vi "Startup.vi"(5 "DAQ":refnum<class "DAQ.lvclass">, 6 "DataQueues":refnum<class "DataQueues.lvclass">, 7 "Application":refnum<class "Application.lvclass">, 8 "error in (no error)":errorcluster, 9 "Config":refnum<class "Config.lvclass">=refnum, 10 "Sequencer":refnum<class "Sequencer.lvclass">=refnum, 11 "LogEngine":refnum<class "LogEngine.lvclass">) -> (0 "error out":errorcluster, 3 "LogEngine.lvclass":refnum<class "LogEngine.lvclass">)   [LabVIEW 2022 SP3, in "LogEngine.lvclass"]
doc: "Developed by Kevin Thompson\nkevin@thompsonengineering.net\n\nCopyright 2018-2020\nThompson Engineering, LLC"
uses:
  LogEngine.lvclass
  LogEngine.lvclass/LogEngine.ctl
  Data Types/TD Logger State Data--cluster.ctl
  Data Types/TD Logger State--enum.ctl
  Support/DataQueues/DataQueues.lvclass
  DAQ/DAQ.lvclass
  Data Types/Dependency--cluster.ctl
  Config/Config.lvclass
  Application/Application.lvclass
  Sequencer/Sequencer.lvclass
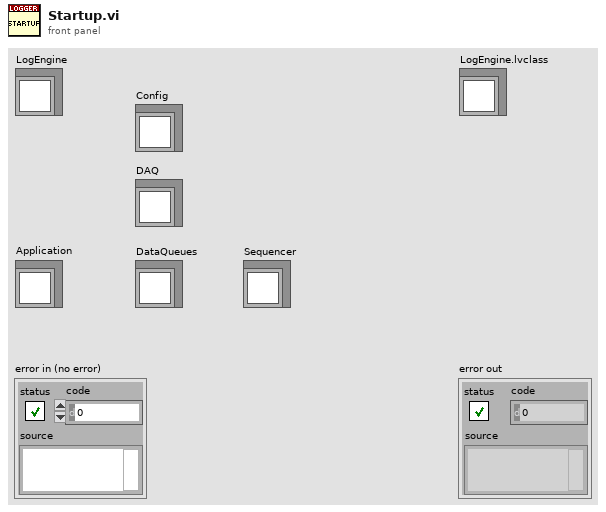
[diagram p1: front panel]
types:
  T1 = typedef "LogEngine.lvclass/Dependency--cluster.ctl" = cluster{"DataQueues":refnum<class "DataQueues.lvclass">, "DAQ":refnum<class "DAQ.lvclass">}
  T2 = typedef "LogEngine.lvclass/TD Logger State Data--cluster.ctl" = cluster{"Logger State":T3, "TDMS Logging State":T3, "LogFile path":path, "TDMS File path":path, "vData":variant}
  T3 = typedef "LogEngine.lvclass/TD Logger State--enum.ctl" = enum16{"Unknown", "Logging", "NotLogging", "Error"}
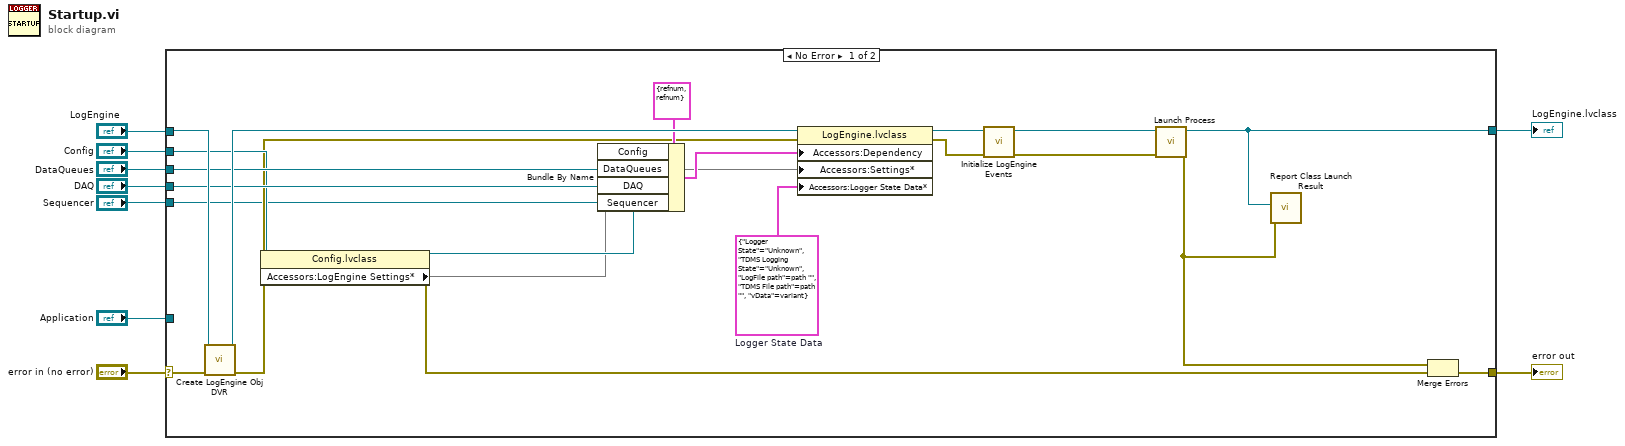
[diagram p0: block diagram]
diagram:
  n1 = case shown="No Error" "error in (no error)" {
    selector: "error in (no error)" -> [w28 w32]
    tunnel: [w30 w32] -> w8
    tunnel: [w12 w31] -> w6
    tunnel: "LogEngine" -> [w27 w31]
    tunnel: "Application" -> [_ _]
    tunnel: "DataQueues" -> [w20 _]
    tunnel: "DAQ" -> [w19 _]
    tunnel: "Config" -> [w17 _]
    tunnel: "Sequencer" -> [w10 _]
    frame No Error {
      w22 = T2 {"Logger State"=enum."Unknown", "TDMS Logging State"=enum."Unknown", "LogFile path"=path "", "TDMS File path"=path "", "vData"=variant}  # Logger State Data
      n2 = call "Create LogEngine Obj DVR.vi"("error in (no error)"=w28, "LogEngine.lvclass"=w27) -> ("error out"=w14:errorcluster, "LogEngine.lvclass"=w26:refnum<class "LogEngine.lvclass">)  [unwired: 8 in]
      n3 = property class="Config.lvclass"(reference=w17, error in=w14) -> (reference out=w16:refnum<class "Config.lvclass">, error out=w13:errorcluster, "Accessors:LogEngine Settings*"=w15)
      n4 = Bundle By Name(cluster=T1 {"DataQueues"=refnum, "DAQ"=refnum} ("Dependency"), "Config"=w16, "DataQueues"=w20, "DAQ"=w19, "Sequencer"=w10) -> (w18:T1)
      n5 = property class="LogEngine.lvclass"(reference=w26, error in=w14, "Accessors:Dependency"=w18, "Accessors:Settings*"=w15, "Accessors:Logger State Data*"=w22) -> (reference out=w25:refnum<class "LogEngine.lvclass">, error out=w29:errorcluster)
      n6 = call "Initialize LogEngine Events.vi"("error in (no error)"=w29, "LogEngine.lvclass"=w25) -> ("error out"=w23:errorcluster, "LogEngine.lvclass"=w24:refnum<class "LogEngine.lvclass">)  [unwired: 8 in]
      n7 = call "Launch Process.vi"("error in (no error)"=w23, "LogEngine.lvclass"=w24) -> ("error out"=w11:errorcluster, "LogEngine.lvclass"=w12:refnum<class "LogEngine.lvclass">)  [unwired: 8 in]
      n8 = call "Report Class Launch Result.vi"("Object"=w12, "error in (no error)"=w11) -> ()  [unwired: 8 in, 1 out]
      n9 = Merge Errors(w11, w13) -> (w30:errorcluster)
    }
    frame Error {
    }
  }
  "error out" <- w8
  "LogEngine.lvclass" <- w6
